vi "Save datapoint.vi"(7 "Use second SMUs":bool, 8 "error in (no error)":errorcluster, 9 "Data in":T1, 10 "Instruments":T2, 11 "graph data in":cluster{"Array":dbl[], "Array":dbl[]}[](array[cluster])) -> (0 "error out":errorcluster, 1 "Is complete":bool, 2 "Data out":T1, 3 "Progress %":dbl(slide) caption="Horizontal Pointer Slide" scale=0.0..100.0, 5 "Graph data out":cluster{"Array":dbl[], "Array":dbl[]}[](array[cluster]))   [LabVIEW 2021]
uses:
  controls/Data.ctl
  <vilib>/GPower/Math/Library/Percent/PercentT/PTI32.vi
  <vilib>/GPower/Math/GPMath.lvlib
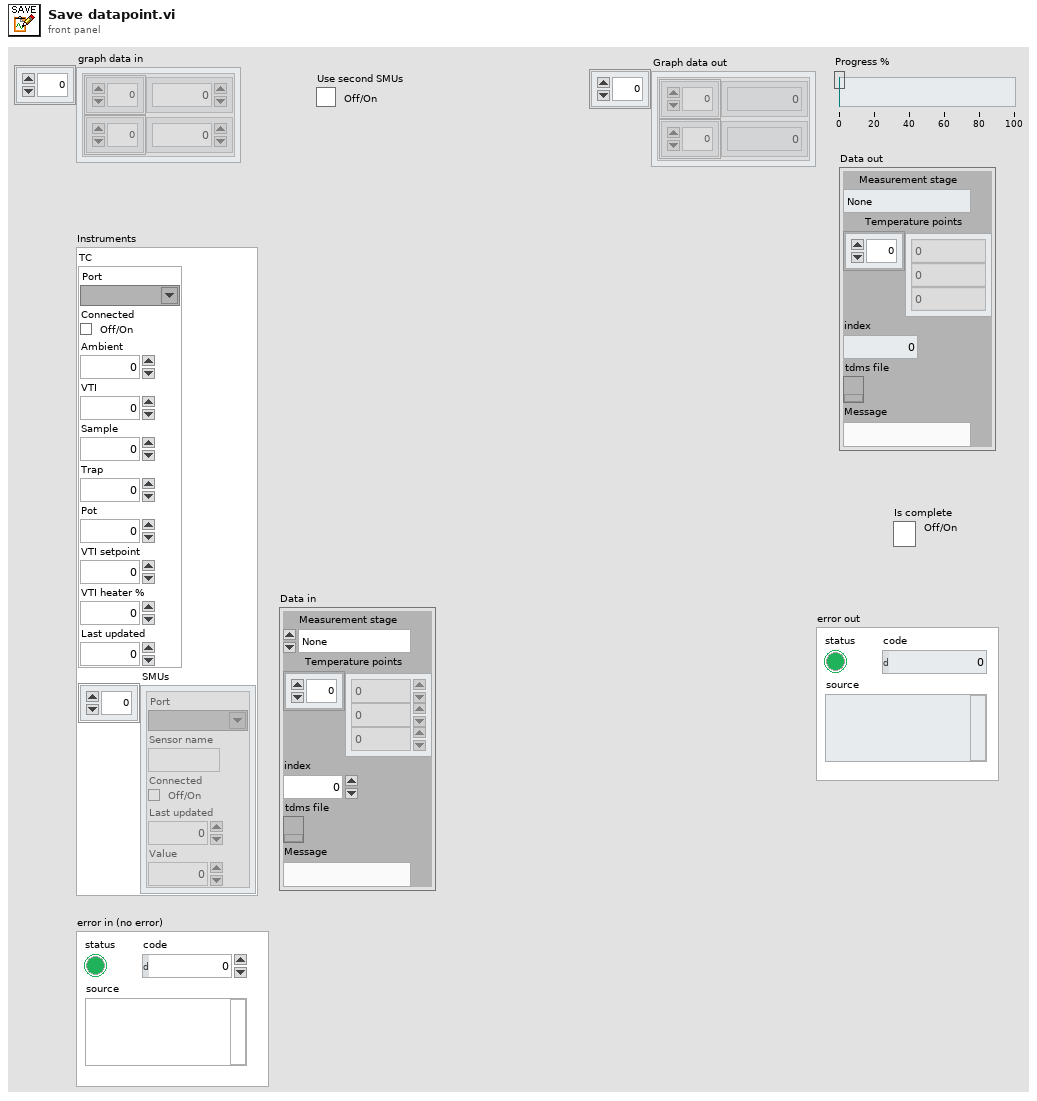
[diagram p1: front panel]
types:
  T1 = typedef "Data.ctl" = cluster{"Measurement stage":enum16{"None", "Wait to start", "Stage 1", "Interstage", "Stage 2", "Stopping"}, "Temperature points":dbl[], "index":i32, "tdms file":refnum<k34>, "Message":string}
  T2 = cluster{"TC":cluster{"Port":refnum<visa-resource-name>, "Connected":bool, "Ambient":dbl, "VTI":dbl, "Sample":dbl, "Trap":dbl, "Pot":dbl, "VTI setpoint":dbl, "VTI heater %":dbl, "Last updated":dbl}, "SMUs":cluster{"Port":refnum<visa-resource-name>, "Sensor name":string, "Connected":bool, "Last updated":dbl, "Value":dbl}[]}
  T3 = cluster{"Port":refnum<visa-resource-name>, "Sensor name":string, "Connected":bool, "Last updated":dbl, "Value":dbl}[]
  T4 = enum16{"None", "Wait to start", "Stage 1", "Interstage", "Stage 2", "Stopping"}
  T5 = cluster{"Port":refnum<visa-resource-name>, "Sensor name":string, "Connected":bool, "Last updated":dbl, "Value":dbl}
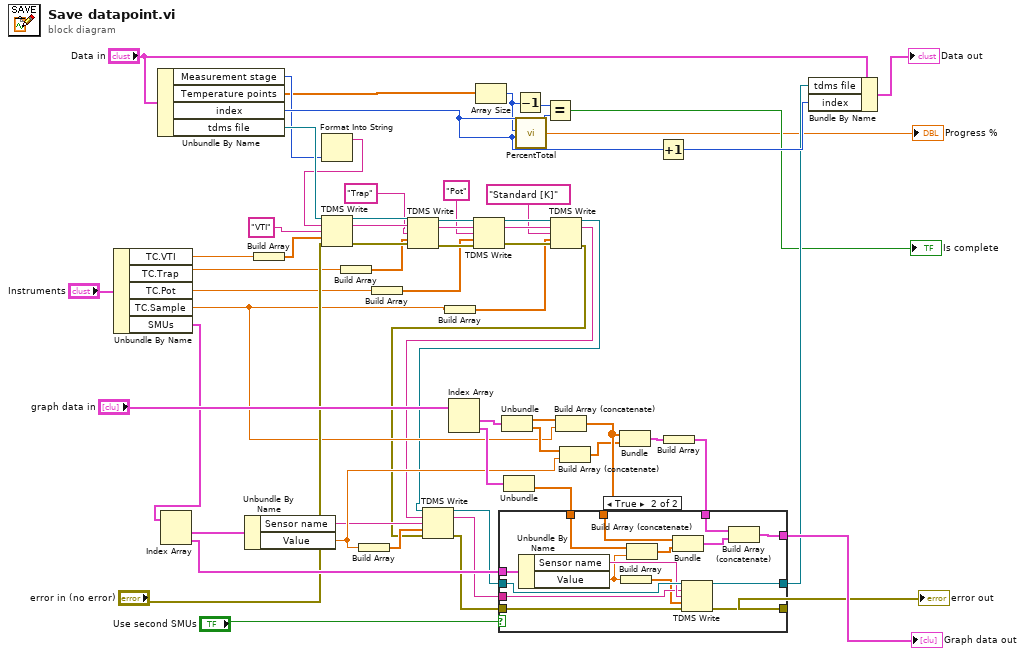
[diagram p0: block diagram]
diagram:
  n1 = Unbundle By Name("Instruments") -> ("TC.VTI"=w14:dbl, "TC.Trap"=w12:dbl, "TC.Pot"=w11:dbl, "TC.Sample"=w4:dbl, "SMUs"=w34:T3)
  n2 = Unbundle By Name("Data in") -> ("Measurement stage"=w31:T4, "Temperature points"=w29:dbl[], "index"=w44:i32, "tdms file"=w33:refnum<k34>)
  n3 = Index Array(array=w34) -> (element #1=w35:T5, element #2=w47:T5)  [unwired: 2 in]
  n4 = Unbundle By Name(w35) -> ("Sensor name"=w39:string, "Value"=w57:dbl)
  n5 = Build Array(w14) -> (w51:dbl[])
  n6 = Format Into String(w31) -> (resulting string=w30:string)  [unwired: 3 in, 1 out]
  n7 = TDMS Write(0:w33, 5:w30, 7:"VTI", 9:w51, 11:"error in (no error)") -> (4:w23:refnum<k34>, 6:w22:string, 15:w21:errorcluster)  [unwired: 1 in, 1 out]
  n8 = Build Array(w12) -> (w9:dbl[])
  n9 = Build Array(w57) -> (w50:dbl[])
  n10 = Build Array(w11) -> (w8:dbl[])
  n11 = TDMS Write(0:w23, 5:w22, 7:"Trap", 9:w9, 11:w21) -> (4:w20:refnum<k34>, 6:w19:string, 15:w18:errorcluster)  [unwired: 1 in, 1 out]
  n12 = Build Array(w4) -> (w6:dbl[])
  n13 = Index Array(array="graph data in") -> (element #1=w54:cluster{"Array":dbl[], "Array":dbl[]}, element #2=w60:cluster{"Array":dbl[], "Array":dbl[]})  [unwired: 2 in]
  n14 = TDMS Write(0:w20, 5:w19, 7:"Pot", 9:w8, 11:w18) -> (4:w17:refnum<k34>, 6:w16:string, 15:w15:errorcluster)  [unwired: 1 in, 1 out]
  n15 = Array Size(array=w29) -> (size(s)=w26:i32)
  n16 = Unbundle(w54) -> ("Array"=w55:dbl[], "Array"=w56:dbl[])
  n17 = Unbundle(w60) -> ("Array"=w61:dbl[])  [unwired: 1 out]
  n18 = Decrement(x=w26) -> (x-1=w25:i32)
  n19 = call-poly <vilib>:"PercentTotal.vi"("b"=w44, "a"=w26) -> ("b % total of a"=→"Progress %":dbl)  [unwired: 4 in]
  n20 = Equal?(x=w25, y=w44) -> (x = y?=→"Is complete":bool)
  n21 = TDMS Write(0:w17, 5:w16, 7:"Standard [K]", 9:w6, 11:w15) -> (4:w1:refnum<k34>, 6:w2:string, 15:w3:errorcluster)  [unwired: 1 in, 1 out]
  n22 = TDMS Write(0:w1, 5:w2, 7:w39, 9:w50, 11:w3) -> (4:w36:refnum<k34>, 6:w37:string, 15:w38:errorcluster)  [unwired: 1 in, 1 out]
  n23 = Build Array (concatenate)(w55, w4) -> (w59:dbl[])
  n24 = Build Array (concatenate)(w56, w57) -> (w58:dbl[])
  n25 = Bundle(w59, w58) -> (w48:cluster{dbl[], dbl[]})  [unwired: 1 in]
  n26 = Increment(x=w44) -> (x+1=w45:i32)
  n27 = Build Array(w48) -> (w49:cluster{dbl[], dbl[]}[])
  n28 = case shown="True" "Use second SMUs" {
    tunnel: w36 -> [w63 w79]
    tunnel: w37 -> [_ w76]
    tunnel: w38 -> [w64 w78]
    tunnel: [w64 w75] -> w40
    tunnel: [w63 w74] -> w43
    tunnel: w47 -> [_ w73]
    tunnel: [w62 w72] -> w52
    tunnel: w49 -> [w62 w70]
    tunnel: w59 -> [_ w71]
    tunnel: w61 -> [_ w66]
    frame False {
    }
    frame True {
      n29 = Unbundle By Name(w73) -> ("Sensor name"=w77:string, "Value"=w65:dbl)
      n30 = Build Array(w65) -> (w69:dbl[])
      n31 = Build Array (concatenate)(w66, w65) -> (w67:dbl[])
      n32 = Bundle(w71, w67) -> (w68:cluster{dbl[], dbl[]})  [unwired: 1 in]
      n33 = TDMS Write(0:w79, 5:w76, 7:w77, 9:w69, 11:w78) -> (4:w74:refnum<k34>, 15:w75:errorcluster)  [unwired: 1 in, 2 out]
      n34 = Build Array (concatenate)(w70, w68) -> (w72:cluster{dbl[], dbl[]}[])
    }
  }
  "Graph data out" <- w52
  "error out" <- w40
  n35 = Bundle By Name(cluster="Data in", "tdms file"=w43, "index"=w45) -> (→"Data out":T1)
